vi "Append Watermark Text.vi"(0 "PDF Report IN":T22(xcontrol), 2 "Watermark Text":T1={"Text "="CONFIDENTIAL", "Opacity (%)"=10.0, "Position"={"Position"=enum."Center (text section)", "X"=0.0, "Y"=0.0}, "Automatic"=FALSE, "Font"={"Font Name"="", "Size"=-1.0, "Color"=0}, "Alignment"=enum."Left", "Rotate(°)"=0.0}, 11 "error in (no error)":errorcluster) -> (4 "PDF Report OUT":T22(xcontrol), 15 "error out":errorcluster)   [LabVIEW 2013]
doc: "Appends a <B>watermark</B> (text or image) on each page of the PDF report. \n\n<B>FRANÇAIS</B>\nAjoute un <B>filigrane</B> (texte or image) sur chaque page du rapport PDF. \n\nVersion 1.0\nDeveloped by Jean-Marc Simard\nCopyright © 2010, Exaprom Inc.\nAll rights reserved.\nLicense: BSD\n\nWith iTextSharp Library\n(http://itextsharp.sourceforge.net)"
uses:
  Controls/PDF Report Xcontrol/PDF Report.xctl
  Controls/Watermark Text Cluster.ctl
  Controls/Watermark Position.ctl
  Controls/Font size.ctl
  Controls/Font color.ctl
  Controls/Header footer horiz alignment.ctl
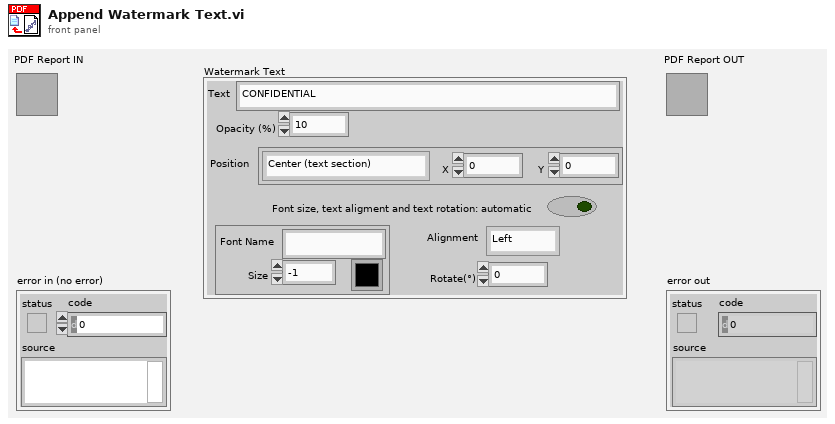
[diagram p1: front panel]
types:
  T1 = typedef "Watermark Text Cluster.ctl" = cluster{"Text ":string, "Opacity (%)":sgl, "Position":cluster{"Position":T2, "X":sgl, "Y":sgl}, "Automatic":bool, "Font":cluster{"Font Name":string, "Size":T3, "Color":T4}, "Alignment":T5, "Rotate(°)":sgl}
  T2 = typedef "Watermark Position.ctl" = enum16{"Absolute", "Center (page)", "Center (text section)"}
  T3 = typedef "Font size.ctl" = sgl
  T4 = typedef "Font color.ctl" = u32
  T5 = typedef "Header footer horiz alignment.ctl" = enum16{"Left", "Center", "Right"}
  T6 = typedef "Font cluster.ctl" = cluster{"Name":string, "Size":T3, "Color":T4, "Style":cluster{"Bold":bool, "Italic":bool, "Underline":bool, "Strikeout":bool}}
  T7 = typedef "Unit.ctl" = enum16{"inch", "mm"}
  T8 = typedef "Paragraphe cluster.ctl" = cluster{" Aligment":T9, "Line spacing":T10}
  T9 = typedef "Texte alignement.ctl" = enum16{"Select", "CENTER", "JUSTIFY", "LEFT", "RIGHT"}
  T10 = typedef "Line spacing.ctl" = enum16{"Select", "1.0", "1.5", "2.0"}
  T11 = typedef "Page dimensions.ctl" = cluster{"Start at page":i32, "Orientation":T12, "widht":sgl, "height":sgl, "Margin left":sgl, "Margin right":sgl, "Margin top":sgl, "Margin bottom":sgl}
  T12 = typedef "Page Orientation.ctl" = enum16{"Portrait", "Landscape"}
  T13 = typedef "Image or Table Caption.ctl" = cluster{"Caption":string, "Separator":string, "Position":enum16{"Above", "Below"}}
  T14 = typedef "Header Footer [ ].ctl" = T15[]
  T15 = typedef "Header Footer cluster.ctl" = cluster{"Start page":i32, "Type":T16, "Alignment":T5, "Vertical Alignement":T17, "Image (%)":sgl, "Page #":T18, "Text":string, "Path":string, "Font":T6, "Font refnum":refnum<k24>, "Line":cluster{"Line":T19, "Thickness (points)":sgl, "Colour":T4}}
  T16 = typedef "Header Footer Type.ctl" = enum16{"Select", "Text", "Text + hyperlink", "Page number", "Image", "Image + hyperlink"}
  T17 = typedef "Cell Vertical alignment.ctl" = enum16{"TOP", "MIDDLE", "BOTTOM"}
  T18 = typedef "Page number.ctl" = cluster{"Text 1":string, "Text 2":string, "Text 3":string}
  T19 = typedef "Header Footer Line.ctl" = enum16{"No line", "Horizontal line"}
  T20 = typedef "Watermark cluster2.ctl" = cluster{"Show? (F)":bool, "Type":enum16{"Image", "Text"}, "Opacity (%)":sgl, "Rotate(°)":sgl, "Position":cluster{"Position":T2, "X":sgl, "Y":sgl}, "Image path":path, "Scaled(%)":sgl, "Image refnum":refnum<k24>, "Text":string, "Font":cluster{"Name":string, "Size":T3, "Color":T4}, "Font refnum":refnum<k24>, "Alignment":T5, "Automatic":bool}
  T21 = typedef "System Fonts.ctl" = cluster{"Font name [ ]":string[], "Font and file names [ ]":cluster{"Font name":string, "File name":string}[]}
  T22 = cluster{"Document":refnum<k24>, "Writer":refnum<k24>, "Default Font":refnum<k24>, "Default Font cluster":T6, "Path":path, "Unit (default = mm)":T7, "Paragraphe cluster":T8, "Pages dimensions [ ]":T11[], "Captions":cluster{"Image":T13, "Image counter":u16, "Table":T13, "Table counter":u16, "Font":T6}, "Header":T14, "Footer":T14, "Watermark ":T20, "Actual VI name":string, "System Fonts":T21}
  T23 = cluster{"Bold":bool, "Italic":bool, "Underline":bool, "Strikeout":bool}
  T24 = cluster{"Font Name":string, "Size":T3, "Color":T4, "Style":cluster{"Bold":bool, "Italic":bool, "Underline":bool, "Strikeout":bool}}
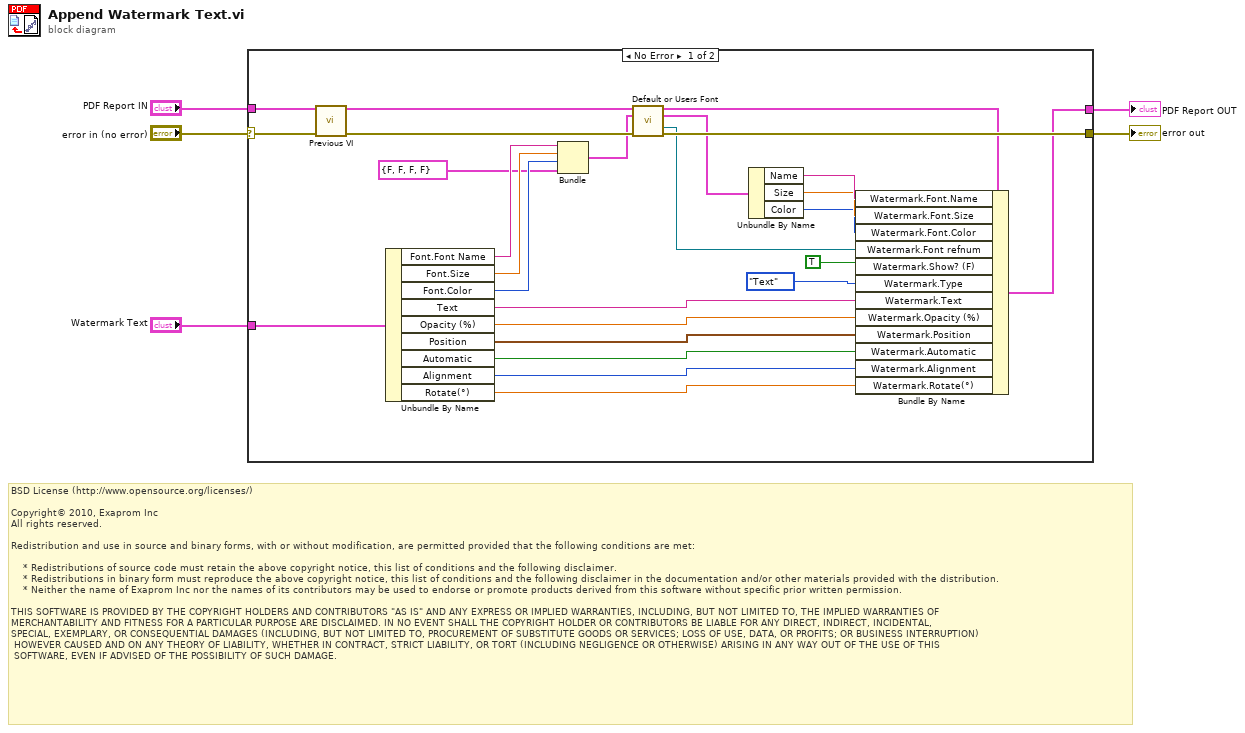
[diagram p0: block diagram]
diagram:
  # "BSD License (http://www.opensource.org/licenses/)\n\nCopyright© 2010, Exaprom Inc\nAll rights reserved.\n\nRedistribution and use in source and binary forms, with or without modification, are permitted provided that the following conditions are met:\n\n    * Redistributions of source code must retain the above copyright notice, this list of conditions and the following disclaimer.\n    * Redistributions in binary form must reproduce the above copyright notice, this list of conditions and the following disclaimer in the documentation and/or other materials provided with the distribution.\n    * Neither the name of Exaprom Inc nor the names of its contributors may be used to endorse or promote products derived from this software without specific prior written permission.\n\nTHIS SOFTWARE IS PROVIDED BY THE COPYRIGHT HOLDERS AND CONTRIBUTORS \"AS IS\" AND ANY EXPRESS OR IMPLIED WARRANTIES, INCLUDING, BUT NOT LIMITED TO, THE IMPLIED WARRANTIES OF \nMERCHANTABILITY AND FITNESS FOR A PARTICULAR PURPOSE ARE DISCLAIMED. IN NO EVENT SHALL THE COPYRIGHT HOLDER OR CONTRIBUTORS BE LIABLE FOR ANY DIRECT, INDIRECT, INCIDENTAL,\nSPECIAL, EXEMPLARY, OR CONSEQUENTIAL DAMAGES (INCLUDING, BUT NOT LIMITED TO, PROCUREMENT OF SUBSTITUTE GOODS OR SERVICES; LOSS OF USE, DATA, OR PROFITS; OR BUSINESS INTERRUPTION)\n HOWEVER CAUSED AND ON ANY THEORY OF LIABILITY, WHETHER IN CONTRACT, STRICT LIABILITY, OR TORT (INCLUDING NEGLIGENCE OR OTHERWISE) ARISING IN ANY WAY OUT OF THE USE OF THIS\n SOFTWARE, EVEN IF ADVISED OF THE POSSIBILITY OF SUCH DAMAGE."
  n1 = case shown="No Error" "error in (no error)" {
    selector: "error in (no error)" -> [w28 w33]
    tunnel: "PDF Report IN" -> [w29 w32]
    tunnel: "Watermark Text" -> [w27 _]
    tunnel: [w30 w32] -> w3
    tunnel: [w31 w33] -> w2
    frame No Error {
      n2 = call "Previous VI.vi"("PDF Report IN"=w29, "error in (no error)"=w28) -> ("PDF Report OUT"=w18:T22, "error out"=w16:errorcluster)  [unwired: 12 out]
      n3 = Unbundle By Name(w27) -> ("Font.Font Name"=w15:string, "Font.Size"=w14:T3, "Font.Color"=w13:T4, "Text"=w24:string, "Opacity (%)"=w23:sgl, "Position"=w22:cluster{"Position":T2, "X":sgl, "Y":sgl}, "Automatic"=w21:bool, "Alignment"=w20:T5, "Rotate(°)"=w19:sgl)
      n4 = Bundle("Font Name"=w15, "Size"=w14, "Color"=w13, "Style"=T23 {"Bold"=FALSE, "Italic"=FALSE, "Underline"=FALSE, "Strikeout"=FALSE}) -> (w11:T24)  [unwired: 1 out]
      n5 = call "Default or Users Font.vi"("PDF Report"=w18, "Font"=w11, "error in (no error)"=w16) -> ("PDF Report duplicate"=w17:T22, "Font OUT"=w10:T6, "Font Ref"=w6:refnum<k24>, "error out"=w31:errorcluster)  [unwired: 9 out]
      n6 = Unbundle By Name(w10) -> ("Name"=w9:string, "Size"=w8:T3, "Color"=w7:T4)
      n7 = Bundle By Name(cluster=w17, "Watermark.Font.Name"=w9, "Watermark.Font.Size"=w8, "Watermark.Font.Color"=w7, "Watermark.Font refnum"=w6, "Watermark.Show? (F)"=TRUE ("Watermark .Show? (F)"), "Watermark.Type"=enum16{"Image", "Text"}."Text" ("Watermark .Type"), "Watermark.Text"=w24, "Watermark.Opacity (%)"=w23, "Watermark.Position"=w22, "Watermark.Automatic"=w21, "Watermark.Alignment"=w20, "Watermark.Rotate(°)"=w19) -> (w30:T22)
    }
    frame Error {
    }
  }
  "PDF Report OUT" <- w3
  "error out" <- w2
